vi "R1Initialize.vi"(8 "error in (no error)":errorcluster) -> (0 "error out":errorcluster)   [LabVIEW 2016]
uses:
  R1Controls/R1SBR_SetParams.ctl
  Controls/pH_SetParams Standard.ctl
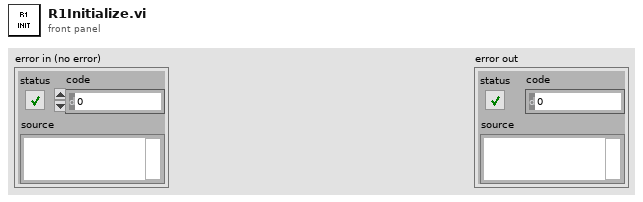
[diagram p1: front panel]
types:
  T1 = cluster{"Set Point, mg/L":dbl, "Tolerance, mg/L":dbl, "N2 Valve Gain":dbl, "Air Valve Gain":dbl}
  T2 = typedef "pH_SetParams Standard.ctl" = cluster{"Set Point":dbl, "Tolerance":dbl, "Pump Time On, secs":dbl}
  T3 = typedef "R1SBR_SetParams.ctl" = cluster{"Phase":string, "Time, min":dbl, "SBR_Manual":cluster{"Media Pump":bool, "Water Pump":bool, "Gas Pump":bool, "Effluent Pump":bool}}[]
  T4 = cluster{"Media Pump":bool, "Water Pump":bool, "Gas Pump":bool, "Effluent Pump":bool}
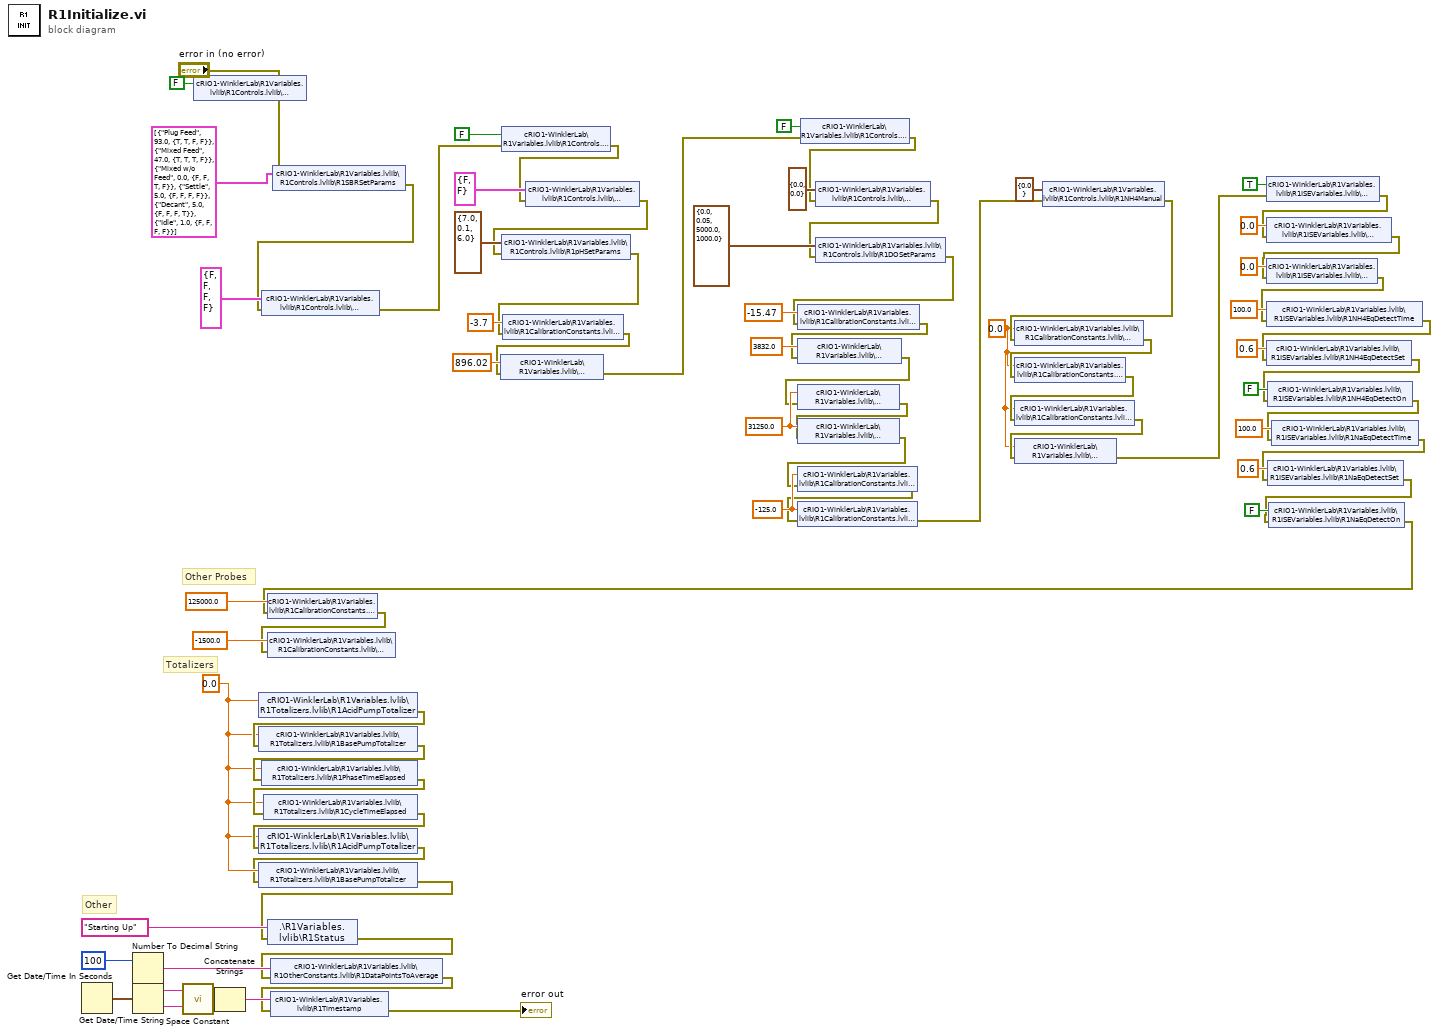
[diagram p0: block diagram]
diagram:
  w20 = 0.0 ("R1NH4Intercept")
  w30 = 0.0 ("R1PhaseTimeElapsed")
  w62 = 31250.0 ("R1AirSlope")
  w63 = -125.0 ("R1N2Intercept")
  # "Totalizers"
  # "Other Probes"
  # "Other"
  n1 = Get Date/Time In Seconds() -> (seconds since 1Jan1904=w39:timestamp)
  n2 = Number To Decimal String(number=100 ("R1DataPointsToAverage")) -> (decimal integer string=w69:string)  [unwired: 1 in]
  n3 = Get Date/Time String(seconds (now)=w39) -> (date string=w27:string, time string=w38:string)  [unwired: 2 in]
  n4 = call <vilib>:"Space Constant.vi"() -> ("String"=w37:string)
  n5 = shared-variable "cRIO1-WinklerLab\\R1Variables.lvlib\\R1Controls.lvlib\\R1SBRSwitch"(FALSE ("R1SBRSwitch")) -> ()  [unwired: 1 in, 1 out]
  n6 = Concatenate Strings(w27, w37, w38) -> (w35:string)
  n7 = shared-variable "cRIO1-WinklerLab\\R1Variables.lvlib\\R1Totalizers.lvlib\\R1AcidPumpTotalizer"(w30) -> (error out=w32:errorcluster)  [unwired: 1 in]
  n8 = shared-variable "cRIO1-WinklerLab\\R1Variables.lvlib\\R1Totalizers.lvlib\\R1BasePumpTotalizer"(w30, error in=w32) -> (error out=w33:errorcluster)
  n9 = shared-variable "cRIO1-WinklerLab\\R1Variables.lvlib\\R1Totalizers.lvlib\\R1PhaseTimeElapsed"(w30, error in=w33) -> (error out=w40:errorcluster)
  n10 = shared-variable "cRIO1-WinklerLab\\R1Variables.lvlib\\R1Totalizers.lvlib\\R1CycleTimeElapsed"(w30, error in=w40) -> (error out=w31:errorcluster)
  n11 = shared-variable "cRIO1-WinklerLab\\R1Variables.lvlib\\R1Totalizers.lvlib\\R1AcidPumpTotalizer"(w30, error in=w31) -> (error out=w29:errorcluster)
  n12 = shared-variable "cRIO1-WinklerLab\\R1Variables.lvlib\\R1Totalizers.lvlib\\R1BasePumpTotalizer"(w30, error in=w29) -> (error out=w28:errorcluster)
  n13 = shared-variable ".\\R1Variables.lvlib\\R1Status"("Starting Up" ("R1Status"), error in=w28) -> (error out=w42:errorcluster)
  n14 = shared-variable "cRIO1-WinklerLab\\R1Variables.lvlib\\R1OtherConstants.lvlib\\R1DataPointsToAverage"(w69, error in=w42) -> (error out=w34:errorcluster)
  n15 = shared-variable "cRIO1-WinklerLab\\R1Variables.lvlib\\R1Timestamp"(w35, error in=w34) -> (error out=→"error out":errorcluster)
  n16 = shared-variable "cRIO1-WinklerLab\\R1Variables.lvlib\\R1Controls.lvlib\\R1SBRSetParams"(T3 [{"Phase"="Plug Feed", "Time, min"=93.0, "SBR_Manual"={"Media Pump"=TRUE, "Water Pump"=TRUE, "Gas Pump"=FALSE, "Effluent Pump"=FALSE}}, {"Phase"="Mixed Feed", "Time, min"=47.0, "SBR_Manual"={"Media Pump"=TRUE, "Water Pump"=TRUE, "Gas Pump"=TRUE, "Effluent Pump"=FALSE}}, {"Phase"="Mixed w/o Feed", "Time, min"=0.0, "SBR_Manual"={"Media Pump"=FALSE, "Water Pump"=FALSE, "Gas Pump"=TRUE, "Effluent Pump"=FALSE}}, {"Phase"="Settle", "Time, min"=5.0, "SBR_Manual"={"Media Pump"=FALSE, "Water Pump"=FALSE, "Gas Pump"=FALSE, "Effluent Pump"=FALSE}}, {"Phase"="Decant", "Time, min"=5.0, "SBR_Manual"={"Media Pump"=FALSE, "Water Pump"=FALSE, "Gas Pump"=FALSE, "Effluent Pump"=TRUE}}, {"Phase"="Idle", "Time, min"=1.0, "SBR_Manual"={"Media Pump"=FALSE, "Water Pump"=FALSE, "Gas Pump"=FALSE, "Effluent Pump"=FALSE}}] ("R1SBR_SetParams 2"), error in="error in (no error)") -> (error out=w58:errorcluster)
  n17 = shared-variable "cRIO1-WinklerLab\\R1Variables.lvlib\\R1Controls.lvlib\\R1SBRManual"(T4 {"Media Pump"=FALSE, "Water Pump"=FALSE, "Gas Pump"=FALSE, "Effluent Pump"=FALSE} ("R1SBR_Manual"), error in=w58) -> (error out=w57:errorcluster)
  n18 = shared-variable "cRIO1-WinklerLab\\R1Variables.lvlib\\R1Controls.lvlib\\R1pHSwitch"(FALSE ("R1pHSwitch"), error in=w57) -> (error out=w56:errorcluster)
  n19 = shared-variable "cRIO1-WinklerLab\\R1Variables.lvlib\\R1Controls.lvlib\\R1pHManual"(cluster{"Acid Pump":bool, "Base Pump":bool} {"Acid Pump"=FALSE, "Base Pump"=FALSE} ("R1pHManual"), error in=w56) -> (error out=w55:errorcluster)
  n20 = shared-variable "cRIO1-WinklerLab\\R1Variables.lvlib\\R1Controls.lvlib\\R1pHSetParams"(T2 {"Set Point"=7.0, "Tolerance"=0.1, "Pump Time On, secs"=6.0} ("R1pHSetParams"), error in=w55) -> (error out=w54:errorcluster)
  n21 = shared-variable "cRIO1-WinklerLab\\R1Variables.lvlib\\R1CalibrationConstants.lvlib\\R1pHIntercept"(-3.7 ("R12pHInt"), error in=w54) -> (error out=w51:errorcluster)
  n22 = shared-variable "cRIO1-WinklerLab\\R1Variables.lvlib\\R1CalibrationConstants.lvlib\\R1pHSlope"(896.02 ("R1pHSlope"), error in=w51) -> (error out=w52:errorcluster)
  n23 = shared-variable "cRIO1-WinklerLab\\R1Variables.lvlib\\R1Controls.lvlib\\R1pHSwitch"(FALSE ("R1pHSwitch"), error in=w52) -> (error out=w50:errorcluster)
  n24 = shared-variable "cRIO1-WinklerLab\\R1Variables.lvlib\\R1Controls.lvlib\\R1DOManual"(cluster{"Air MFC":dbl, "N2 MFC":dbl} {"Air MFC"=0.0, "N2 MFC"=0.0} ("R1DOManual"), error in=w50) -> (error out=w49:errorcluster)
  n25 = shared-variable "cRIO1-WinklerLab\\R1Variables.lvlib\\R1Controls.lvlib\\R1DOSetParams"(T1 {"Set Point, mg/L"=0.0, "Tolerance, mg/L"=0.05, "N2 Valve Gain"=5000.0, "Air Valve Gain"=1000.0} ("R1DOSetParams"), error in=w49) -> (error out=w48:errorcluster)
  n26 = shared-variable "cRIO1-WinklerLab\\R1Variables.lvlib\\R1CalibrationConstants.lvlib\\R1DOIntercept"(-15.47 ("R1DOInt"), error in=w48) -> (error out=w47:errorcluster)
  n27 = shared-variable "cRIO1-WinklerLab\\R1Variables.lvlib\\R1CalibrationConstants.lvlib\\R1DOSlope"(3832.0 ("R1DOSlope"), error in=w47) -> (error out=w46:errorcluster)
  n28 = shared-variable "cRIO1-WinklerLab\\R1Variables.lvlib\\R1CalibrationConstants.lvlib\\R1N2Slope"(w62, error in=w46) -> (error out=w45:errorcluster)
  n29 = shared-variable "cRIO1-WinklerLab\\R1Variables.lvlib\\R1CalibrationConstants.lvlib\\R1AirSlope"(w62, error in=w45) -> (error out=w44:errorcluster)
  n30 = shared-variable "cRIO1-WinklerLab\\R1Variables.lvlib\\R1CalibrationConstants.lvlib\\R1AirIntercept"(w63, error in=w44) -> (error out=w43:errorcluster)
  n31 = shared-variable "cRIO1-WinklerLab\\R1Variables.lvlib\\R1CalibrationConstants.lvlib\\R1N2Intercept"(w63, error in=w43) -> (error out=w25:errorcluster)
  n32 = shared-variable "cRIO1-WinklerLab\\R1Variables.lvlib\\R1Controls.lvlib\\R1NH4Manual"(cluster{"NH4 Pump Flowrate, ml/min":dbl} {"NH4 Pump Flowrate, ml/min"=0.0} ("R1NH4Manual"), error in=w25) -> (error out=w24:errorcluster)
  n33 = shared-variable "cRIO1-WinklerLab\\R1Variables.lvlib\\R1CalibrationConstants.lvlib\\R1NH4Intercept"(w20, error in=w24) -> (error out=w21:errorcluster)
  n34 = shared-variable "cRIO1-WinklerLab\\R1Variables.lvlib\\R1CalibrationConstants.lvlib\\R1NH4Slope"(w20, error in=w21) -> (error out=w23:errorcluster)
  n35 = shared-variable "cRIO1-WinklerLab\\R1Variables.lvlib\\R1CalibrationConstants.lvlib\\R1NaIntercept"(w20, error in=w23) -> (error out=w22:errorcluster)
  n36 = shared-variable "cRIO1-WinklerLab\\R1Variables.lvlib\\R1CalibrationConstants.lvlib\\R1NaSlope"(w20, error in=w22) -> (error out=w10:errorcluster)
  n37 = shared-variable "cRIO1-WinklerLab\\R1Variables.lvlib\\R1ISEVariables.lvlib\\R1NH4NaOn"(TRUE ("R1NH4NaOn"), error in=w10) -> (error out=w9:errorcluster)
  n38 = shared-variable "cRIO1-WinklerLab\\R1Variables.lvlib\\R1ISEVariables.lvlib\\R1NH4NaConc"(0.0 ("R1NH4NaConc"), error in=w9) -> (error out=w8:errorcluster)
  n39 = shared-variable "cRIO1-WinklerLab\\R1Variables.lvlib\\R1ISEVariables.lvlib\\R1NH4NaCF"(0.0 ("R1NH4NaCF"), error in=w8) -> (error out=w7:errorcluster)
  n40 = shared-variable "cRIO1-WinklerLab\\R1Variables.lvlib\\R1ISEVariables.lvlib\\R1NH4EqDetectTime"(100.0 ("R1NH4EqDetectTime"), error in=w7) -> (error out=w6:errorcluster)
  n41 = shared-variable "cRIO1-WinklerLab\\R1Variables.lvlib\\R1ISEVariables.lvlib\\R1NH4EqDetectSet"(0.6 ("R1NH4EqDetectSet"), error in=w6) -> (error out=w5:errorcluster)
  n42 = shared-variable "cRIO1-WinklerLab\\R1Variables.lvlib\\R1ISEVariables.lvlib\\R1NH4EqDetectOn"(FALSE ("R1NH4EqDetectOn"), error in=w5) -> (error out=w4:errorcluster)
  n43 = shared-variable "cRIO1-WinklerLab\\R1Variables.lvlib\\R1ISEVariables.lvlib\\R1NaEqDetectTime"(100.0 ("R1NaEqDetectTime"), error in=w4) -> (error out=w3:errorcluster)
  n44 = shared-variable "cRIO1-WinklerLab\\R1Variables.lvlib\\R1ISEVariables.lvlib\\R1NaEqDetectSet"(0.6 ("R1NaEqDetectSet"), error in=w3) -> (error out=w2:errorcluster)
  n45 = shared-variable "cRIO1-WinklerLab\\R1Variables.lvlib\\R1ISEVariables.lvlib\\R1NaEqDetectOn"(FALSE ("R1NaEqDetectOn"), error in=w2) -> (error out=w1:errorcluster)
  n46 = shared-variable "cRIO1-WinklerLab\\R1Variables.lvlib\\R1CalibrationConstants.lvlib\\R1ORPSlope"(125000.0 ("R1ORPSlope"), error in=w1) -> (error out=w41:errorcluster)
  n47 = shared-variable "cRIO1-WinklerLab\\R1Variables.lvlib\\R1CalibrationConstants.lvlib\\R1ORPIntercept"(-1500.0 ("R1ORPIntercept"), error in=w41) -> ()  [unwired: 1 out]
